vi "S2DS_Create File name (SubVI).vi"(11 "User info":string[](array[string])) -> (3 "File name":string)   [LabVIEW 2025]
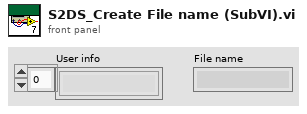
[diagram p1: front panel]
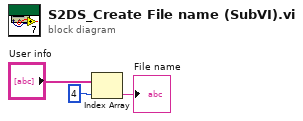
[diagram p0: block diagram]
diagram:
  n1 = Index Array(array="User info", index=4) -> (element=→"File name":string)
